vi "check if there is pulse.vi"() -> ()   [LabVIEW 2014]
panel:
  in  "y":u32
  out "Array 2":bool[](array[boolean])
  out "Numeric Control":u32
  in  "Array":bool[](array[boolean])
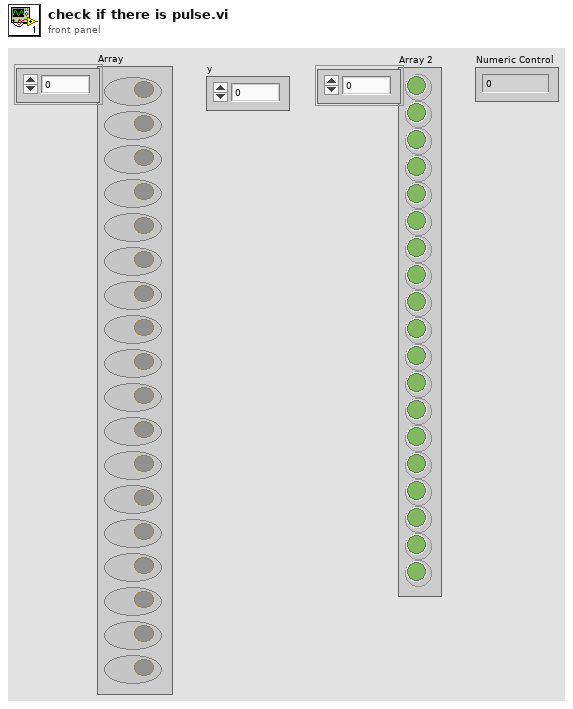
[diagram p1: front panel]
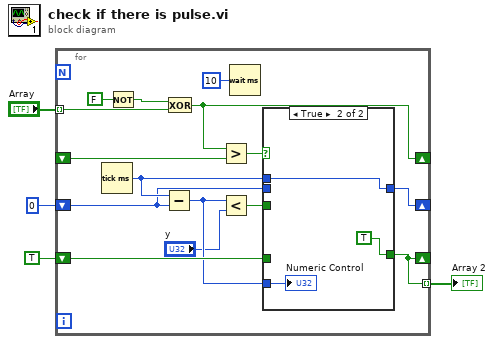
[diagram p0: block diagram]
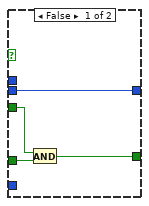
[diagram p2: hidden frame]
diagram:
  n1 = for {
    tunnel: "Array" -> [w17] mode=indexing
    shift-right: [w16] -> _
    shift-left: _ -> [w15]
    shift-right: [w11] -> _
    shift-left: u32 0 ("Tick Count(Ticks)") -> [w12]
    shift-right: [w9] -> _
    shift-left: TRUE ("x") -> [w10]
    tunnel: [w9] -> w1 mode=indexing
    n2 = Tick Count (ms)() -> (millisecond timer value=w13:u32)
    n3 = Not(x=FALSE) -> (.not. x?=w19:bool)
    n4 = Subtract(x=w13, y=w12) -> (x-y=w8:u32)
    n5 = Exclusive Or(1:w17, 2:w19) -> (0:w16:bool)
    n6 = Greater?(x=w16, y=w15) -> (0:w14:bool)
    n7 = Less?(x=w8, y="y") -> (x < y?=w6:bool)
    n8 = Wait (ms)(milliseconds to wait=u32 10 ("millisecond multiple")) -> ()  [unwired: 1 out]
    n9 = case shown="True" w14 {
      tunnel: w13 -> [_ w26]
      tunnel: w8 -> [_ w25]
      tunnel: w12 -> [w23 _]
      tunnel: [w23 w26] -> w11
      tunnel: w10 -> [w22 _]
      tunnel: [w21 TRUE] -> w9
      tunnel: w6 -> [w20 _]
      frame False {
        n10 = And(x=w20, y=w22) -> (x .and. y?=w21:bool)
      }
      frame True {
        "Numeric Control" <- w25
      }
    }
  }
  "Array 2" <- w1
